vi "Simulated VeriStand Engine.Interface.Write.Stop.vi"(8 "error in (no error)":errorcluster, 10 "stop":bool, 11 "Simulated VeriStand Engine Interface in":refnum<class "Simulated VeriStand Engine.Interface.lvclass">) -> (0 "error out":errorcluster, 3 "Simulated VeriStand Engine Interface out":refnum<class "Simulated VeriStand Engine.Interface.lvclass">)   [LabVIEW 2016, in "Simulated VeriStand Engine.Interface.lvclass"]
uses:
  Simulated VeriStand Engine.Interface.lvclass
  Simulated VeriStand Engine.Interface.lvclass/Simulated VeriStand Engine.Interface.ctl
  Source/Submodules/Memory/Source/Classes/Pointer/Memory.Pointer.lvclass/Memory.Pointer.ctl
  Accessors/Simulated VeriStand Engine.Interface.Get Control Pointers.vi
  Source/Submodules/Memory/Source/Classes/Pointer/Memory.Pointer.Write.Safe.0D.Bool.vi
  Source/Submodules/Memory/Source/Classes/Pointer/Memory.Pointer.Write.Unsafe.0D.Bool.vi
  Source/Submodules/Memory/Source/Classes/Pointer/Memory.Pointer.Parameter Check.Null Pointer.vi
  Source/Submodules/Memory/Source/Classes/Pointer/Memory.Pointer.Parameter Check.Subset.vi
  Source/Submodules/Memory/Source/Classes/Pointer/Memory.Pointer.Get Address.vi
  Source/Submodules/Memory/Source/Classes/Pointer/Memory.Pointer.Errors.vi
  Source/Submodules/Memory/Source/Classes/Pointer/Memory.Pointer.Errors.Null Pointer.vi
  Source/Submodules/Memory/Source/Classes/Pointer/Memory.Pointer.Errors.Out of Bounds.vi
  Source/Submodules/Memory/Source/Classes/Pointer/Memory.Pointer.Get Size.vi
  Source/Submodules/Memory/Source/Classes/Pointer/Memory.Pointer.Errors.Create Error.vi
  Source/Submodules/Memory/Source/Submodules/SEH/Source/VIs/Static Error Handling.Source Buffer.Write.String.vi
  Source/Submodules/Memory/Source/Classes/Pointer/Memory.Pointer.Errors.Write Pointer Size.vi
  Source/Submodules/Memory/Source/Submodules/SEH/Source/VIs/Static Error Handling.Source Buffer.Write.Numeric.Scalar.Base10.vi
  Source/Submodules/Memory/Source/Submodules/SEH/Source/VIs/Static Error Handling.Source Buffer.Write.Numeric.Scalar.Base10 (U64).vi
  Source/Submodules/Memory/Source/Submodules/SEH/Source/VIs/Static Error Handling.Error Cluster Constant.vi
  Source/Submodules/Memory/Source/Submodules/SEH/Source/VIs/Static Error Handling.Error Cluster Constant (256B).vi
  Source/Submodules/Memory/Source/Submodules/SEH/Source/VIs/Static Error Handling.Parameters.Status.Set.vi
  Source/Submodules/Memory/Source/Submodules/SEH/Source/VIs/Static Error Handling.Parameters.Code.Set.vi
  Source/Submodules/Memory/Source/Submodules/SEH/Source/VIs/Static Error Handling.Parameters.VI Source.Set.vi
  Source/Submodules/Memory/Source/Constants/Memory.Constants.vi
  Source/Submodules/Memory/Source/Constants/Memory.Constants.Library Name.vi
  Source/Submodules/Memory/Source/Classes/Pointer/Memory.Pointer.Errors.Get Info.vi
  Source/Submodules/Memory/Source/Classes/Internal/Memory.Pointer.Internal.lvclass
  C:/Git/SourceTree/DSF/Source/Submodules/Memory/Source/Classes/Pointer/Memory.Pointer.lvclass
  Source/Submodules/Memory/Source/Classes/Pointer/Memory.Pointer.lvclass
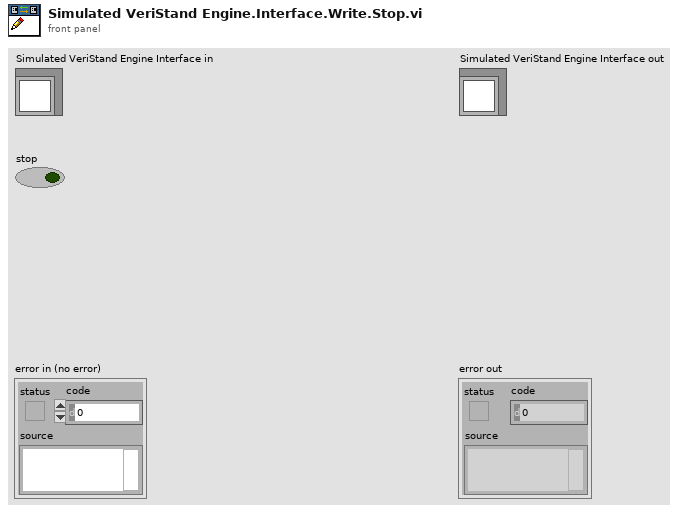
[diagram p1: front panel]
types:
  T1 = typedef "Simulated VeriStand Engine.Interface.lvclass/Simulated VeriStand Engine.Interface.Pointers.Control.ctl" = cluster{"Stop":refnum<class "Memory.Pointer.Internal.lvclass">, "Target Period (µs)":refnum<class "Memory.Pointer.Internal.lvclass">}
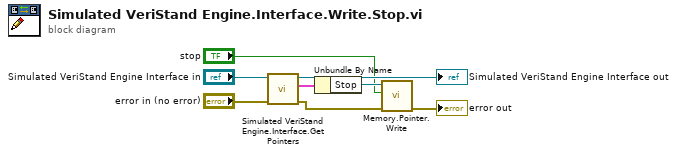
[diagram p0: block diagram]
diagram:
  n1 = call-poly "Simulated VeriStand Engine.Interface.Get Pointers.vi"("error in (no error)"="error in (no error)", "Simulated VeriStand Engine Interface in"="Simulated VeriStand Engine Interface in") -> ("error out"=w6:errorcluster, "Control Pointers"=w8:T1, "Simulated VeriStand Engine Interface out"=→"Simulated VeriStand Engine Interface out":refnum<class "Simulated VeriStand Engine.Interface.lvclass">)  [unwired: 7 in]
  n2 = Unbundle By Name(w8) -> ("Stop"=w7:refnum<class "Memory.Pointer.Internal.lvclass">)
  n3 = call-poly "Memory.Pointer.Write.vi"("error in (no error)"=w6, "value"="stop", "pointer in"=w7) -> ("error out"=→"error out":errorcluster)  [unwired: 5 in, 3 out]
